vi "E364x Select Voltage.vi"(7 "Output Enabled (F: Off)":bool=TRUE, 8 "error in":errorcluster, 9 "Level (0.0 Volts)":dbl=5.0, 10 "Output":string, 11 "VISA in":refnum<visa-resource-name>) -> (0 "error out":errorcluster, 3 "VISA Out":refnum<visa-resource-name>)   [LabVIEW 2017]
uses:
  Agilent E364X Series/Agilent E364X Series.lvlib
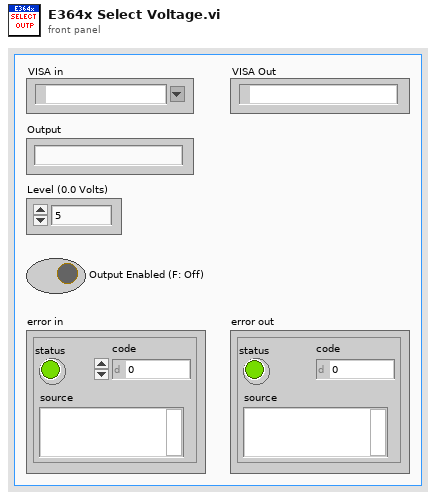
[diagram p1: front panel]
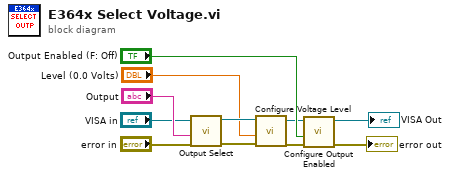
[diagram p0: block diagram]
diagram:
  n1 = call "Output Select.vi"("error in (no error)"="error in", "Instrument Select (Output 1)"="Output", "VISA resource name"="VISA in") -> ("error out"=w6:errorcluster, "VISA resource name out"=w7:refnum<visa-resource-name>)  [unwired: 7 in]
  n2 = call "Configure Voltage Level.vi"("error in (no error)"=w6, "Level (0.0 Volts)"="Level (0.0 Volts)", "VISA resource name"=w7) -> ("error out"=w8:errorcluster, "VISA resource name out"=w10:refnum<visa-resource-name>)  [unwired: 7 in]
  n3 = call "Configure Output Enabled.vi"("error in (no error)"=w8, "Output Enabled (F: Off)"="Output Enabled (F: Off)", "VISA resource name"=w10) -> ("error out"=→"error out":errorcluster, "VISA resource name out"=→"VISA Out":refnum<visa-resource-name>)  [unwired: 7 in]
